vi "testTx.vi"() -> ()   [LabVIEW 2013]
uses:
  lv_lib/CHR34XXX.lvlib
panel:
  in  "Mode":u8
  in  "pstRsdcb":T1
  in  "通道号":u8 max=23 step=1
  out "devId":i32
  out "Exit":bool
  in  "退出":bool
  in  "(10us)":u32=100000
  in  "定时发送":bool
  out "RxFlag":bool
  in  "发送":bool
  out "布尔":bool
  in  "TxData(Hex)":string
  in  "通道号":u8 max=23 step=1
  # "Mode：通道模式，0 表示 232 模式，1 表示 422 模式，2 表示 485 模式 \nBaudRate：波特率\nRS232：75~500Kbps\nRS422/485：75~2.4Mbps\nByteSize：数据位长度，取值范围为 5~8\nStopBits：停止位个数，取值范围为 0~2\n取值为 0 时，表示 1 位停止位(ByteSize 取值为 5~8)\n取值为 1 时，表示 1.5 位停止位(ByteSize 取值为 5)\n取值为 2 时，表示 2 位停止位(ByteSize 取值为 6~8)\nParity：校验方式，取值范围为 0~4\n0：无校验，1：奇校验，2：偶校验，3：Mark 校验，4：Space 校验"
  # "勾选发送周期可设置定时发送模式"
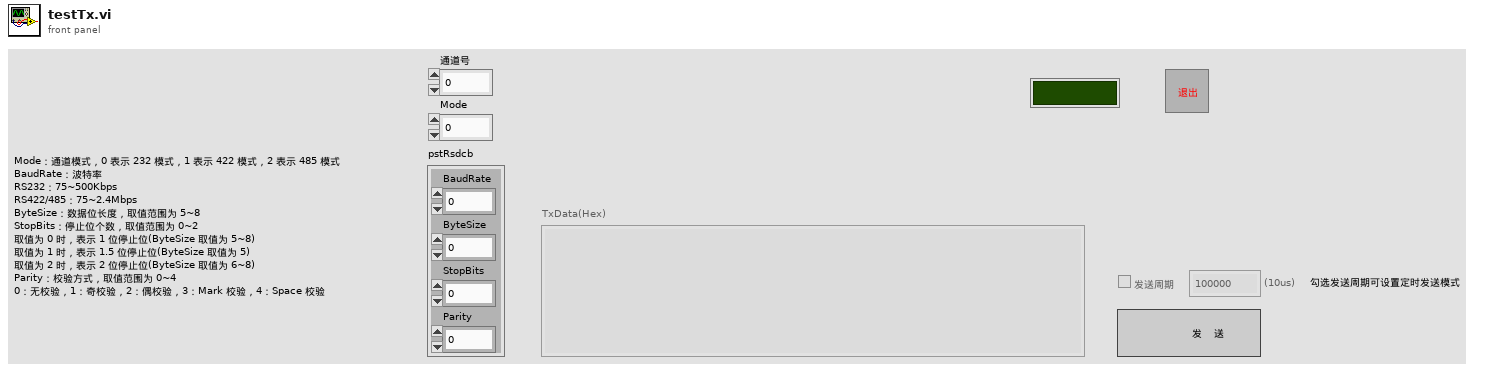
[diagram p1: front panel]
types:
  T1 = cluster{"BaudRate":u32, "ByteSize":u32, "StopBits":u32, "Parity":u32}
  T2 = enum8{"Enabled", "Disabled", "Disabled and Grayed Out"}
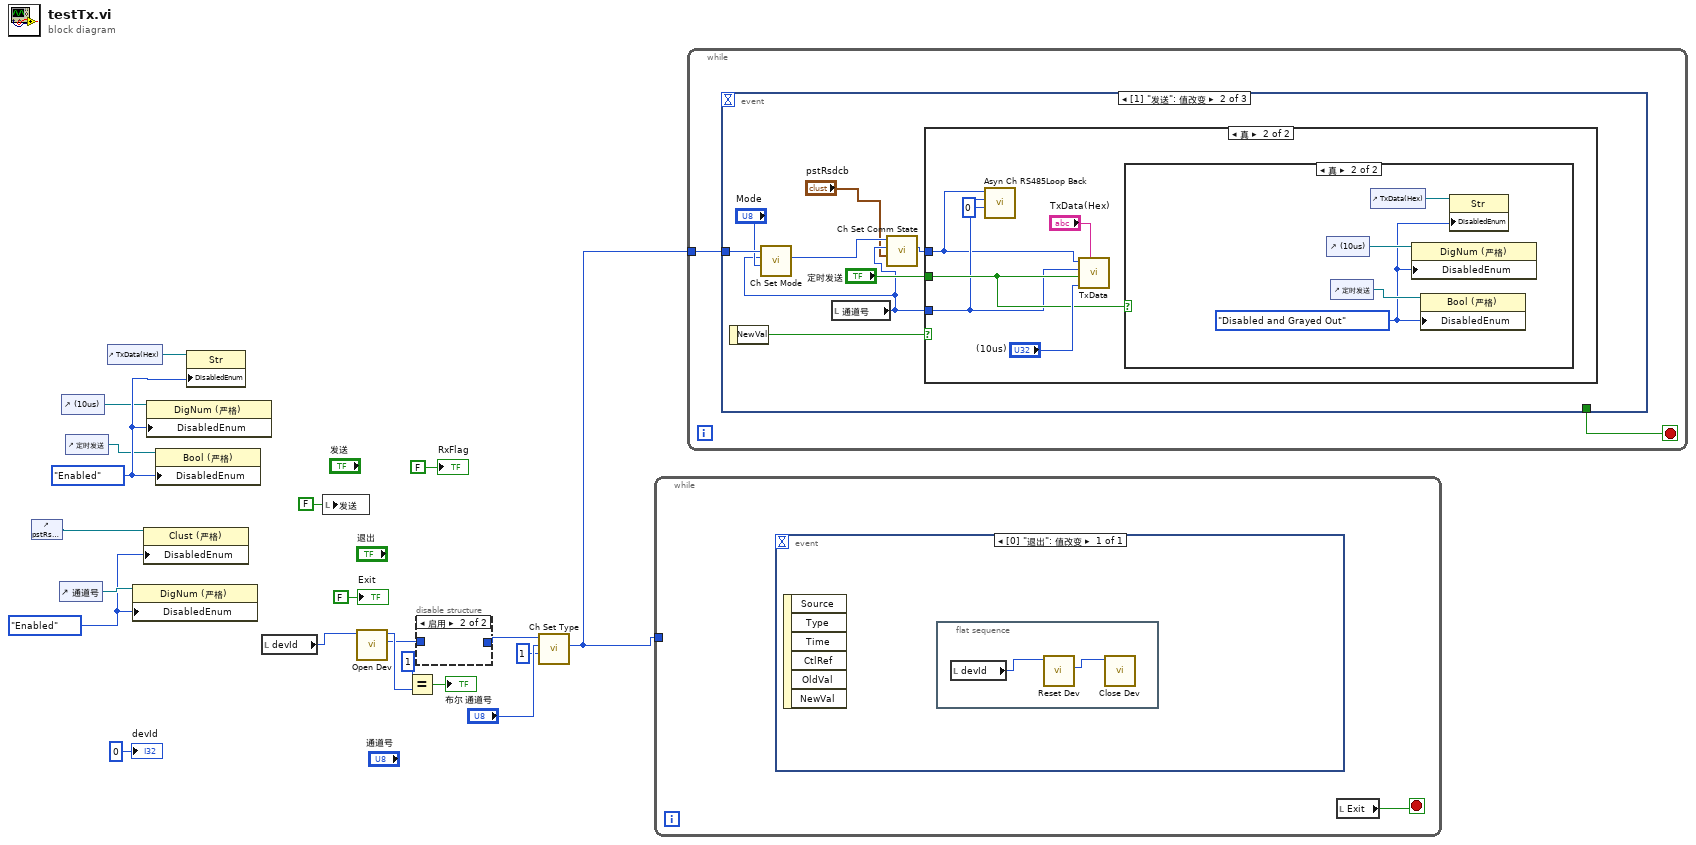
[diagram p0: block diagram]
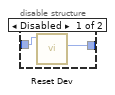
[diagram p2: hidden frame]
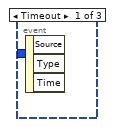
[diagram p3: hidden frame]
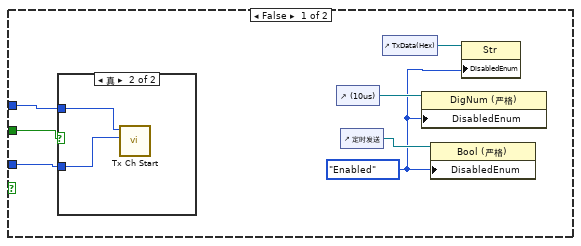
[diagram p4: hidden frame]
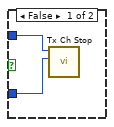
[diagram p5: hidden frame]
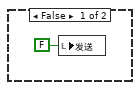
[diagram p6: hidden frame]
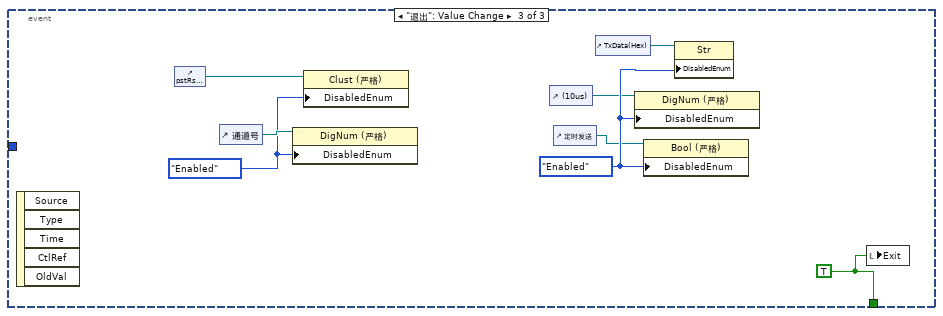
[diagram p7: hidden frame]
diagram:
  w13 = T2."Enabled" ("禁用")
  w14 = T2."Enabled" ("禁用")
  n1 = control-ref of="pstRsdcb"() -> (w9:refnum<vi>)
  n2 = control-ref of="通道号"() -> (w15:refnum<vi>)
  n3 = control-ref of="(10us)"() -> (w10:refnum<vi>)
  n4 = control-ref of="定时发送"() -> (w11:refnum<vi>)
  n5 = control-ref of="TxData(Hex)"() -> (w12:refnum<vi>)
  n6 = property class="DigNum (严格)"(reference=w15, "DisabledEnum"=w14) -> ()  [unwired: 1 in, 2 out]
  n7 = property class="Clust (严格)"(reference=w9, "DisabledEnum"=w14) -> ()  [unwired: 1 in, 2 out]
  n8 = property class="DigNum (严格)"(reference=w10, "DisabledEnum"=w13) -> ()  [unwired: 1 in, 2 out]
  n9 = property class="Bool (严格)"(reference=w11, "DisabledEnum"=w13) -> ()  [unwired: 1 in, 2 out]
  n10 = property class="Str"(reference=w12, "DisabledEnum"=w13) -> ()  [unwired: 1 in, 2 out]
  n11 = local read "devId"() -> (w8:i32)
  n12 = local write "发送"(FALSE ("发送")) -> ()
  n13 = call "Open Dev.vi"("devId in"=w8) -> ("devId out"=w2:i32, "function return"=w17:i32)  [unwired: 9 in]
  n14 = Equal?(x=1, y=w17) -> (x = y?=→"布尔":bool)
  n15 = disable-structure shown="启用" {
    disable-tunnel: w2 -> [w22 _]
    disable-tunnel: [w21 _] -> w1
    frame Disabled {
      n16 = call "Reset Dev.vi"("devId"=w22) -> ("devId out"=w21:i32)  [unwired: 9 in, 1 out]
    }
    frame Enabled {
    }
  }
  n17 = call "Ch Set Type.vi"("Type"=u8 1, "Channel"="通道号", "devId"=w1) -> ("devId out"=w3:i32)  [unwired: 7 in, 1 out]
  n18 = while {
    tunnel: w3 -> [_]
    stop <- w23 stop-if-true
    n19 = event shown="[0] \"退出\": 值改变" {
      selector: _ -> [_]
      dyn-events: _ -> [_]
      timeout: _ -> [_]
      event "退出": Value Change {
        n20 = event-data() -> ()  [unwired: 1 in, 6 out]
        n21 = flat-sequence {
          frame #0 {
            n22 = local read "devId"() -> (w24:i32)
            n23 = call "Reset Dev.vi"("devId"=w24) -> ("devId out"=w25:i32)  [unwired: 9 in, 1 out]
            n24 = call "Close Dev.vi"("devId"=w25) -> ()  [unwired: 9 in, 2 out]
          }
        }
      }
    }
    n25 = local read "Exit"() -> (w23:bool)
  }
  n26 = while {
    tunnel: w3 -> [w27]
    stop <- w26 stop-if-true
    n27 = event shown="[1] \"发送\": 值改变" {
      selector: _ -> [_ _ _]
      dyn-events: _ -> [_ _ _]
      timeout: _ -> [_ _ _]
      tunnel: w27 -> [_ w32 _]
      tunnel: [_ _ w65] -> w26
      event Timeout {
        n28 = event-data() -> ()  [unwired: 1 in, 3 out]
      }
      event "发送": Value Change {
        n29 = event-data() -> ("NewVal"=w35:bool)  [unwired: 1 in]
        n30 = local read "通道号"() -> (w30:u8)
        n31 = call "Ch Set Mode.vi"("Mode"="Mode", "Channel"=w30, "devId"=w32) -> ("devId out"=w33:i32)  [unwired: 7 in, 1 out]
        n32 = call "Ch Set Comm State.vi"("pstRsdcb"="pstRsdcb", "Channel"=w30, "devId"=w33) -> ("devId out"=w29:i32)  [unwired: 6 in, 2 out]
        n33 = case shown="真" w35 {
          tunnel: w29 -> [w42 w48]
          tunnel: w30 -> [w41 w49]
          tunnel: "定时发送" -> [w40 w50]
          frame False {
            w36 = T2."Enabled" ("禁用")
            n34 = case shown="真" w40 {
              tunnel: w42 -> [w44 w46]
              tunnel: w41 -> [w43 w45]
              frame False {
                n35 = call "Tx Ch Stop.vi"("Channel"=w43, "devId"=w44) -> ()  [unwired: 8 in, 2 out]
              }
              frame True {
                n36 = call "Tx Ch Start.vi"("Channel"=w45, "devId"=w46) -> ()  [unwired: 8 in, 2 out]
              }
            }
            n37 = control-ref of="(10us)"() -> (w39:refnum<vi>)
            n38 = control-ref of="定时发送"() -> (w38:refnum<vi>)
            n39 = control-ref of="TxData(Hex)"() -> (w37:refnum<vi>)
            n40 = property class="DigNum (严格)"(reference=w39, "DisabledEnum"=w36) -> ()  [unwired: 1 in, 2 out]
            n41 = property class="Bool (严格)"(reference=w38, "DisabledEnum"=w36) -> ()  [unwired: 1 in, 2 out]
            n42 = property class="Str"(reference=w37, "DisabledEnum"=w36) -> ()  [unwired: 1 in, 2 out]
          }
          frame True {
            n43 = call "Asyn Ch RS485Loop Back.vi"("Enabled"=0, "Channel"=w49, "devId"=w48) -> ()  [unwired: 7 in, 2 out]
            n44 = call "TxData.vi"("TxData(Hex)"="TxData(Hex)", "Period(10us)"="(10us)", "定时发送"=w50, "通道号"=w49, "Handle"=w48) -> ()  [unwired: 7 in]
            n45 = case shown="真" w50 {
              frame False {
                n46 = local write "发送"(FALSE ("发送")) -> ()
              }
              frame True {
                w54 = T2."Disabled and Grayed Out" ("禁用")
                n47 = control-ref of="(10us)"() -> (w57:refnum<vi>)
                n48 = control-ref of="定时发送"() -> (w56:refnum<vi>)
                n49 = control-ref of="TxData(Hex)"() -> (w55:refnum<vi>)
                n50 = property class="DigNum (严格)"(reference=w57, "DisabledEnum"=w54) -> ()  [unwired: 1 in, 2 out]
                n51 = property class="Bool (严格)"(reference=w56, "DisabledEnum"=w54) -> ()  [unwired: 1 in, 2 out]
                n52 = property class="Str"(reference=w55, "DisabledEnum"=w54) -> ()  [unwired: 1 in, 2 out]
              }
            }
          }
        }
      }
      event "退出": Value Change {
        w62 = T2."Enabled" ("禁用")
        w63 = T2."Enabled" ("禁用")
        w65 = TRUE
        n53 = event-data() -> ()  [unwired: 1 in, 5 out]
        n54 = control-ref of="pstRsdcb"() -> (w58:refnum<vi>)
        n55 = control-ref of="通道号"() -> (w64:refnum<vi>)
        n56 = property class="DigNum (严格)"(reference=w64, "DisabledEnum"=w63) -> ()  [unwired: 1 in, 2 out]
        n57 = property class="Clust (严格)"(reference=w58, "DisabledEnum"=w63) -> ()  [unwired: 1 in, 2 out]
        n58 = control-ref of="(10us)"() -> (w59:refnum<vi>)
        n59 = control-ref of="定时发送"() -> (w60:refnum<vi>)
        n60 = control-ref of="TxData(Hex)"() -> (w61:refnum<vi>)
        n61 = property class="DigNum (严格)"(reference=w59, "DisabledEnum"=w62) -> ()  [unwired: 1 in, 2 out]
        n62 = property class="Bool (严格)"(reference=w60, "DisabledEnum"=w62) -> ()  [unwired: 1 in, 2 out]
        n63 = property class="Str"(reference=w61, "DisabledEnum"=w62) -> ()  [unwired: 1 in, 2 out]
        n64 = local write "Exit"(w65) -> ()
      }
    }
  }
  "RxFlag" <- FALSE ("RxFlag")
  "Exit" <- FALSE ("Exit")
  "devId" <- 0 ("devId")
